vi "Main.vi"() -> ()   [LabVIEW 2022 SP3]
doc: "该范例项目基于标准状态机模板创建，演示用于采集、分析和显示数据的应用程序创建方法。 该应用程序的功能包括：显示配置对话框、在多次执行间保持设置、加载和保存数据，以及导出图像和文本文件。\n\n既不允许在采集过程中更新屏幕，也不允许将数据连续写入磁盘，因此特别适用于快速采集数据。"
uses:
  controls/State.ctl
  controls/Data.ctl
  controls/UI References.ctl
  controls/Graph Data.ctl
  <vilib>/Utility/miscctls.llb/LVAnnotationListTypeDef.ctl
  <vilib>/Utility/miscctls.llb/LVCursorListTypeDef.ctl
  controls/User Specified Data.ctl
  controls/HW Configuration.ctl
  controls/Simulated Signal Type.ctl
  controls/Analysis Configuration.ctl
  controls/New Data Behavior.ctl
  subVIs/Settings Dialog.vi
panel:
  in  "设置":bool
  in  "快照":bool
  in  "分析":bool
  in  "清空":bool
  in  "退出":bool
  in  "采集":bool
  in  "导出":bool
  in  "保存数据":bool
  in  "加载数据":bool
  out "图形":waveform(dbl)[](graph)
  out "状态栏":string
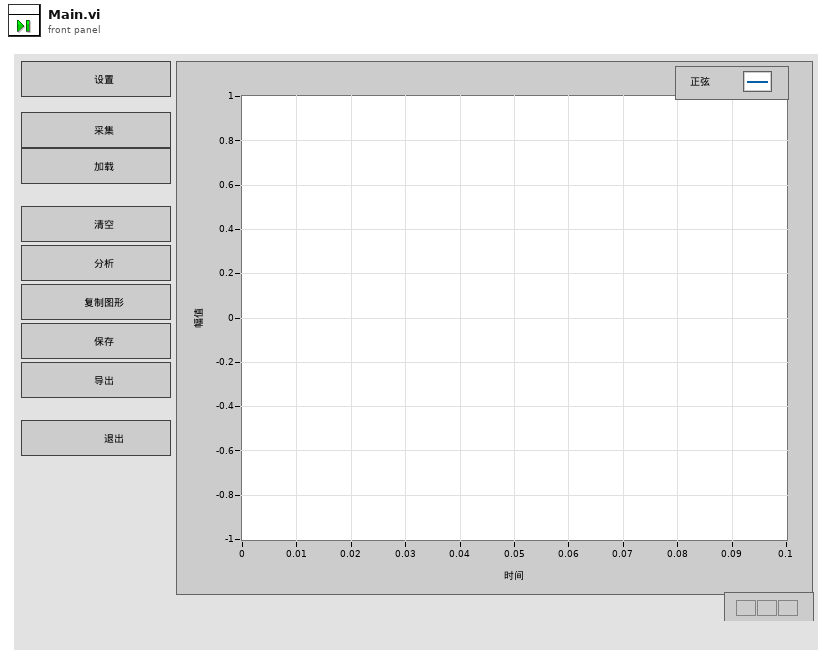
[diagram p1: front panel]
types:
  T1 = typedef "Data.ctl" = cluster{"UI引用":T2, "图形数据":T3, "用户定义":T6}
  T2 = typedef "UI References.ctl" = cluster{"退出引用":refnum<vi>, "保存引用":refnum<vi>, "打开引用":refnum<vi>, "导出引用":refnum<vi>, "采集引用":refnum<vi>, "配置引用":refnum<vi>, "图形引用":refnum<vi>, "清空引用":refnum<vi>, "分析引用":refnum<vi>, "状态引用":refnum<vi>, "快照引用":refnum<vi>}
  T3 = typedef "Graph Data.ctl" = cluster{"数据":waveform(dbl)[], "注释列表":T4, "游标列表":T5, "分析数据":waveform(dbl)[]}
  T4 = typedef "LVAnnotationListTypeDef.ctl" = cluster{"Name":string, "Color":u32, "Style":u8, "Point Style":u8, "Name Visible":bool, "Allow Drag":bool, "Annotation Mode":u32, "Plot":i32, "Index":i32, "Position":cluster{"X":dbl, "Y":dbl}, "X Scale":u32, "Y Scale":u32, "Show Arrow":bool, "Lock Name":bool, "Plot Area":i32, "Label Offset":cluster{"X":dbl, "Y":dbl}}[]
  T5 = typedef "LVCursorListTypeDef.ctl" = cluster{"Name":string, "Color":u32, "Style":u8, "Point Style":u8, "Name Visible":bool, "Allow Drag":bool, "Cursor Mode":u32, "Plot":i32, "Index":i32, "Position":cluster{"X":dbl, "Y":dbl}, "X Scale":u32, "Y Scale":u32, "Watch Plots":i32[], "Watch All Plots":bool, "Plot Area":i32, "Label Offset":cluster{"X":dbl, "Y":dbl}}[]
  T6 = typedef "User Specified Data.ctl" = cluster{"硬件配置":T7, "分析配置":T9, "新采集到数据时如何操作":T10}
  T7 = typedef "HW Configuration.ctl" = cluster{"硬件引用句柄<替换此项>":string, "信号类型<替换该项>":T8}
  T8 = typedef "Simulated Signal Type.ctl" = enum16{"Sine Wave", "Square Wave"}
  T9 = typedef "Analysis Configuration.ctl" = cluster{"统计":bool}
  T10 = typedef "New Data Behavior.ctl" = enum16{"Replace", "Overlay", "Append"}
  T11 = typedef "State.ctl" = enum16{"Initialize", "Wait for Event", "Update UI", "Configure", "Acquire", "Load Data", "Save Data", "Clear Data", "Export Data", "Analyze", "Copy Graph", "Exit"}
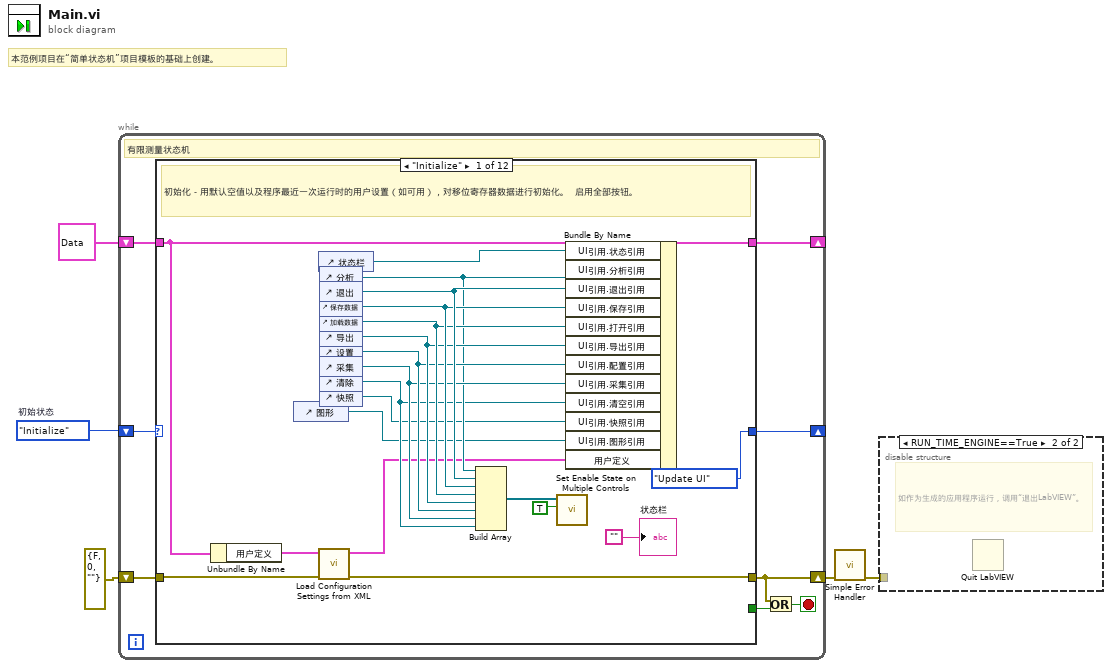
[diagram p0: block diagram]
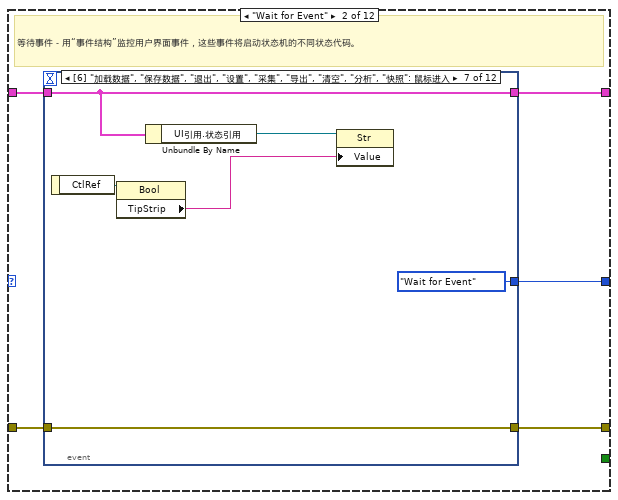
[diagram p3: hidden frame]
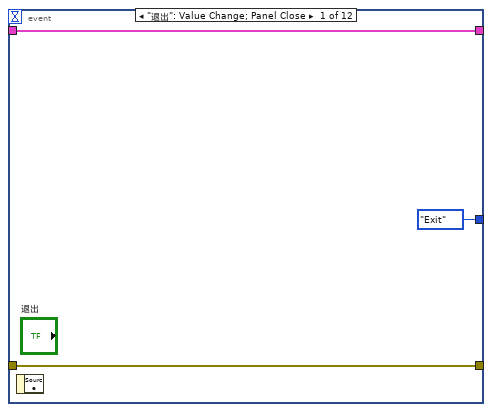
[diagram p4: hidden frame]
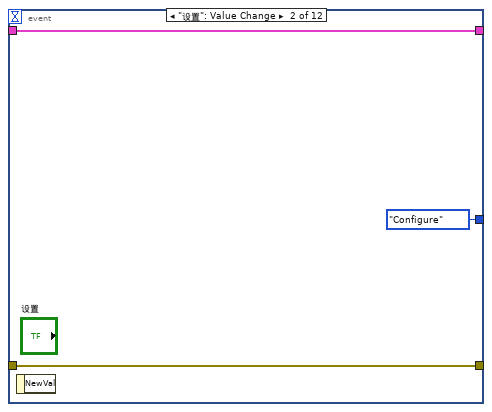
[diagram p5: hidden frame]
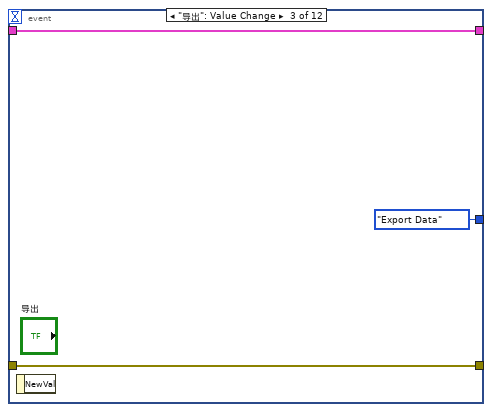
[diagram p6: hidden frame]
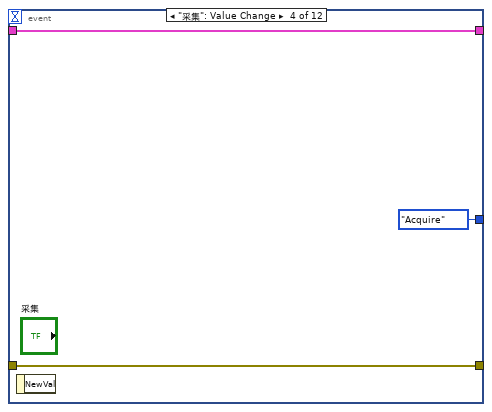
[diagram p7: hidden frame]
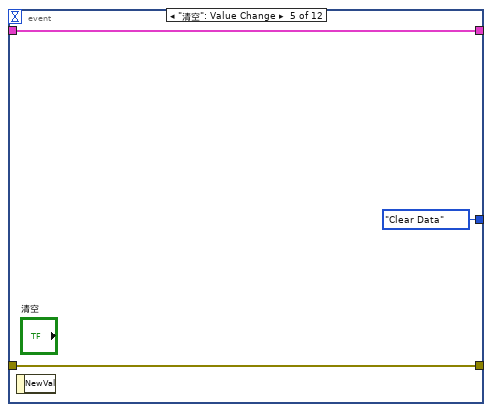
[diagram p8: hidden frame]
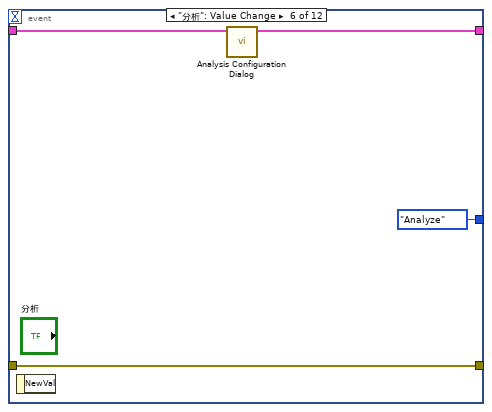
[diagram p9: hidden frame]
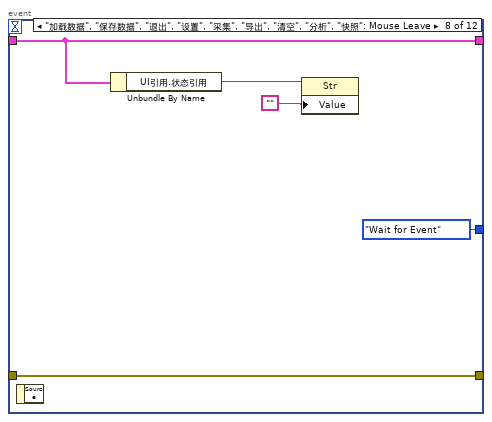
[diagram p10: hidden frame]
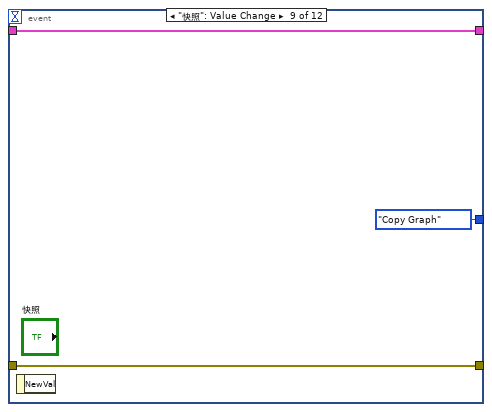
[diagram p11: hidden frame]
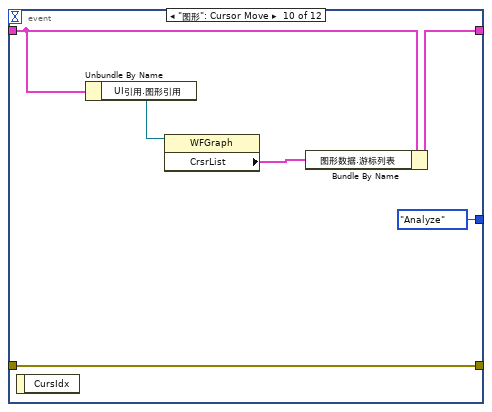
[diagram p12: hidden frame]
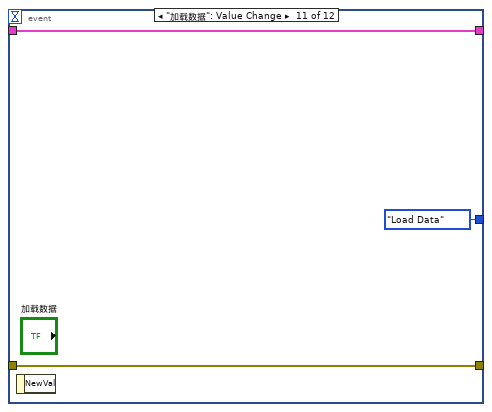
[diagram p13: hidden frame]
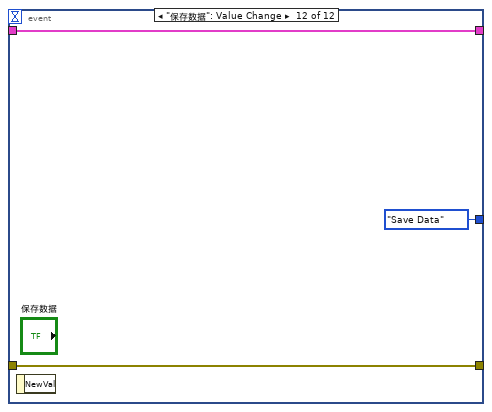
[diagram p14: hidden frame]
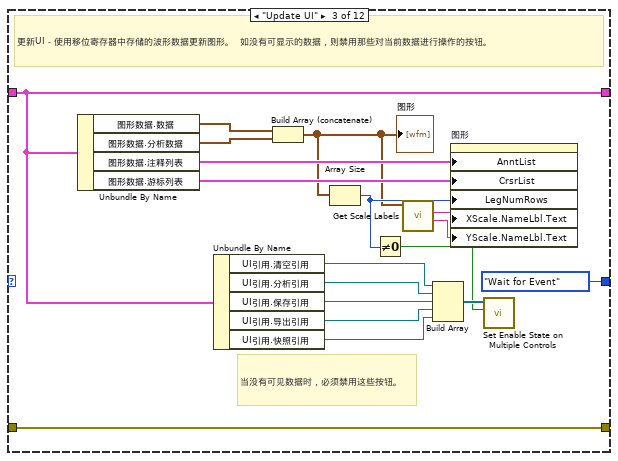
[diagram p15: hidden frame]
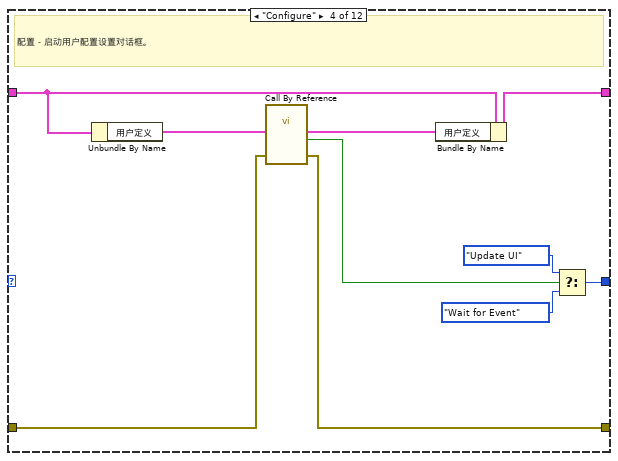
[diagram p16: hidden frame]
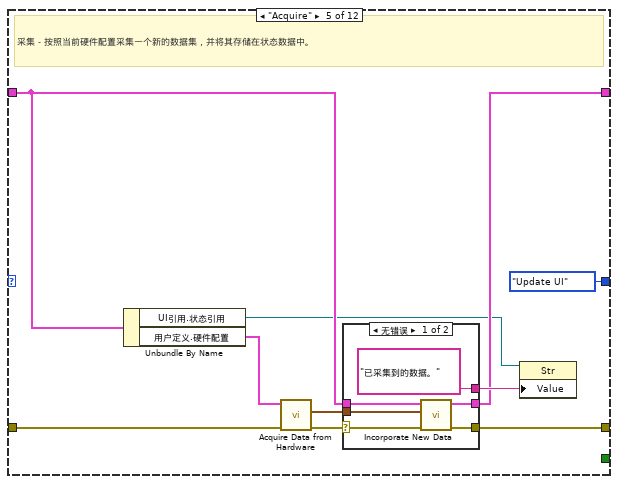
[diagram p17: hidden frame]
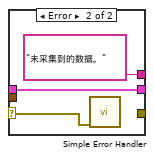
[diagram p18: hidden frame]
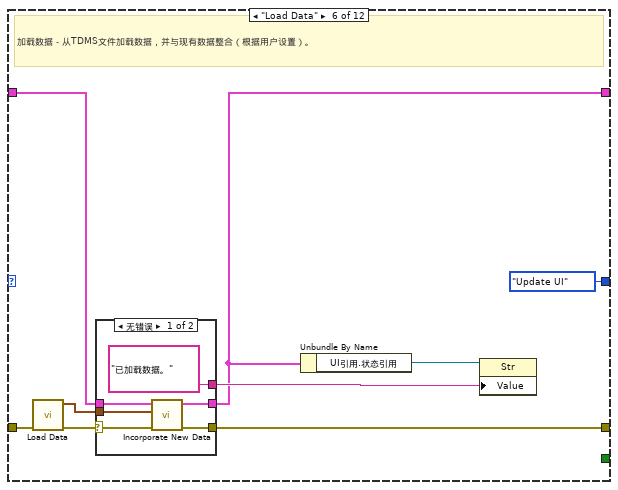
[diagram p19: hidden frame]
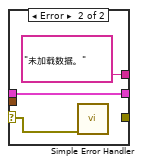
[diagram p20: hidden frame]
diagram:
  w5 = State."Initialize"  # 初始状态
  # "本范例项目在“简单状态机”项目模板的基础上创建。"
  n1 = while {
    shift-right: [w12] -> _
    shift-left: w5 -> [w13]
    shift-right: [w10] -> _
    shift-left: T1 {"UI引用"={"退出引用"=refnum, "保存引用"=refnum, "打开引用"=refnum, "导出引用"=refnum, "采集引用"=refnum, "配置引用"=refnum, "图形引用"=refnum, "清空引用"=refnum, "分析引用"=refnum, "状态引用"=refnum, "快照引用"=refnum}, "图形数据"={"数据"=[], "注释列表"=[], "游标列表"=[], "分析数据"=[]}, "用户定义"={"硬件配置"={"硬件引用句柄<替换此项>"="", "信号类型<替换该项>"=enum."Sine Wave"}, "分析配置"={"统计"=TRUE}, "新采集到数据时如何操作"=enum."Replace"}} ("Data") -> [w11]
    shift-right: [w6] -> w3
    shift-left: errorcluster {"status"=FALSE, "code"=0, "source"=""} ("error constant") -> [w9]
    stop <- w7 stop-if-true
    # "有限测量状态机"
    n2 = case shown="\"Initialize\"" w13 {
      tunnel: [State."Update UI" ("Next State") w39 State."Wait for Event" ("(Value Not Used)") w106 State."Update UI" ("Next State") State."Update UI" ("(Value Not Used)") State."Wait for Event" ("(Value Not Used)") State."Wait for Event" ("(Value Not Used)") State."Update UI" ("(Value Not Used)") State."Update UI" ("(Value Not Used)") State."Wait for Event" ("(Value Not Used)") w194] -> w12
      tunnel: [_ _ _ _ _ _ _ _ _ _ _ w193] -> w8
      tunnel: w11 -> [w25 w38 w99 w112 w118 w140 w153 w165 w176 w179 w185 w191]
      tunnel: [w33 w37 w99 w111 w117 w134 w153 w165 w175 w179 w185 w191] -> w10
      tunnel: w9 -> [w23 w36 w102 w110 w120 w139 w155 w168 w178 w180 w184 w188]
      tunnel: [w22 w35 w102 w109 w113 w138 w151 w162 w178 w180 w183 w187] -> w6
      frame "Initialize" {
        # "初始化－用默认空值以及程序最近一次运行时的用户设置（如可用），对移位寄存器数据进行初始化。  启用全部按钮。"
        n3 = Unbundle By Name(w25) -> ("用户定义"=w24:T6)
        n4 = control-ref of="图形"() -> (w14:refnum<vi>)
        n5 = control-ref of="状态栏"() -> (w20:refnum<vi>)
        n6 = call "Load Configuration Settings from XML.vi"("error in (no error)"=w23, "用户配置输入"=w24) -> ("error out"=w22:cluster{"状态":bool, "代码":i32, "源":string}, "用户配置输出"=w17:T6)  [unwired: 8 in]
        n7 = control-ref of="分析"() -> (w21:refnum<vi>)
        n8 = control-ref of="退出"() -> (w32:refnum<vi>)
        n9 = control-ref of="保存数据"() -> (w31:refnum<vi>)
        n10 = control-ref of="加载数据"() -> (w30:refnum<vi>)
        n11 = control-ref of="导出"() -> (w29:refnum<vi>)
        n12 = control-ref of="设置"() -> (w28:refnum<vi>)
        n13 = control-ref of="采集"() -> (w27:refnum<vi>)
        n14 = control-ref of="清除"() -> (w19:refnum<vi>)
        n15 = control-ref of="快照"() -> (w15:refnum<vi>)
        n16 = Build Array(w21, w32, w31, w30, w29, w28, w27, w19) -> (w26:refnum<vi>[])
        n17 = call "Set Enable State on Multiple Controls.vi"("启用？"=TRUE ("Enable?"), "控件"=w26) -> ()  [unwired: 10 in]
        n18 = Bundle By Name(cluster=w25, "UI引用.状态引用"=w20, "UI引用.分析引用"=w21, "UI引用.退出引用"=w32, "UI引用.保存引用"=w31, "UI引用.打开引用"=w30, "UI引用.导出引用"=w29, "UI引用.配置引用"=w28, "UI引用.采集引用"=w27, "UI引用.清空引用"=w19, "UI引用.快照引用"=w15, "UI引用.图形引用"=w14, "用户定义"=w17) -> (w33:T1)
        "状态栏" <- "" ("Status Bar")
      }
      frame "Wait for Event" {
        # "等待事件－用“事件结构”监控用户界面事件，这些事件将启动状态机的不同状态代码。"
        n19 = event shown="[6] \"加载数据\", \"保存数据\", \"退出\", \"设置\", \"采集\", \"导出\", \"清空\", \"分析\", \"快照\": 鼠标进入" {
          selector: _ -> [_ _ _ _ _ _ _ _ _ _ _ _]
          dyn-events: _ -> [_ _ _ _ _ _ _ _ _ _ _ _]
          timeout: _ -> [_ _ _ _ _ _ _ _ _ _ _ _]
          tunnel: [State."Exit" ("Next State") State."Configure" ("Next State") State."Export Data" ("Next State") State."Acquire" ("Next State") State."Clear Data" ("Next State") State."Analyze" ("Next State") State."Wait for Event" ("Next State") State."Wait for Event" ("Next State") State."Copy Graph" ("Next State") State."Analyze" ("Next State") State."Load Data" ("Next State") State."Save Data" ("Next State")] -> w39
          tunnel: w38 -> [w41 w45 w48 w51 w54 w56 w62 w68 w72 w73 w80 w83]
          tunnel: [w41 w45 w48 w51 w54 w55 w62 w68 w72 w76 w80 w83] -> w37
          tunnel: w36 -> [w40 w44 w47 w50 w53 w58 w64 w69 w71 w78 w79 w82]
          tunnel: [w40 w44 w47 w50 w53 w58 w64 w69 w71 w78 w79 w82] -> w35
          event "退出": Value Change; Panel Close {
            n20 = event-data() -> ()  [unwired: 1 in, 1 out]
          }
          event "设置": Value Change {
            n21 = event-data() -> ()  [unwired: 1 in, 1 out]
          }
          event "导出": Value Change {
            n22 = event-data() -> ()  [unwired: 1 in, 1 out]
          }
          event "采集": Value Change {
            n23 = event-data() -> ()  [unwired: 1 in, 1 out]
          }
          event "清空": Value Change {
            n24 = event-data() -> ()  [unwired: 1 in, 1 out]
          }
          event "分析": Value Change {
            n25 = event-data() -> ()  [unwired: 1 in, 1 out]
            n26 = call "Analysis Configuration Dialog.vi"("数据输入"=w56) -> ("数据输出"=w55:T1)  [unwired: 10 in]
          }
          event "加载数据", "保存数据", "退出", "设置", "采集", "导出", "清空", "分析", "快照": Mouse Enter {
            n27 = event-data() -> ("CtlRef"=w63:refnum<vi>)  [unwired: 1 in]
            n28 = property on="Property Node" class="Bool"(reference=w63) -> ("TipStrip"=w60:string)  [unwired: 1 in, 2 out]
            n29 = Unbundle By Name(w62) -> ("UI引用.状态引用"=w61:refnum<vi>)
            n30 = property on="Property Node" class="Str"(reference=w61, "Value"=w60) -> ()  [unwired: 1 in, 2 out]
          }
          event "加载数据", "保存数据", "退出", "设置", "采集", "导出", "清空", "分析", "快照": Mouse Leave {
            n31 = event-data() -> ()  [unwired: 1 in, 1 out]
            n32 = Unbundle By Name(w68) -> ("UI引用.状态引用"=w67:refnum<vi>)
            n33 = property on="Property Node" class="Str"(reference=w67, "Value"="") -> ()  [unwired: 1 in, 2 out]
          }
          event "快照": Value Change {
            n34 = event-data() -> ()  [unwired: 1 in, 1 out]
          }
          event "图形": Cursor Move {
            n35 = event-data() -> ()  [unwired: 1 in, 1 out]
            n36 = Unbundle By Name(w73) -> ("UI引用.图形引用"=w75:refnum<vi>)
            n37 = property on="Property Node" class="WFGraph"(reference=w75) -> ("CrsrList"=w74:T5)  [unwired: 1 in, 2 out]
            n38 = Bundle By Name(cluster=w73, "图形数据.游标列表"=w74) -> (w76:T1)
          }
          event "加载数据": Value Change {
            n39 = event-data() -> ()  [unwired: 1 in, 1 out]
          }
          event "保存数据": Value Change {
            n40 = event-data() -> ()  [unwired: 1 in, 1 out]
          }
        }
      }
      frame "Update UI" {
        # "当没有可见数据时，必须禁用这些按钮。"
        # "更新UI－使用移位寄存器中存储的波形数据更新图形。  如没有可显示的数据，则禁用那些对当前数据进行操作的按钮。"
        n41 = Unbundle By Name(w99) -> ("图形数据.数据"=w95:waveform(dbl)[], "图形数据.分析数据"=w85:waveform(dbl)[], "图形数据.注释列表"=w100:T4, "图形数据.游标列表"=w96:T5)
        n42 = Unbundle By Name(w99) -> ("UI引用.清空引用"=w91:refnum<vi>, "UI引用.分析引用"=w90:refnum<vi>, "UI引用.保存引用"=w98:refnum<vi>, "UI引用.导出引用"=w88:refnum<vi>, "UI引用.快照引用"=w89:refnum<vi>)
        n43 = Build Array (concatenate)(w95, w85) -> (w93:waveform(dbl)[])
        "图形" <- w93
        n44 = Array Size(array=w93) -> (size(s)=w94:i32)
        n45 = Not Equal To 0?(x=w94) -> (x != 0?=w92:bool)
        n46 = call "Get Scale Labels.vi"("波形数组"=w93) -> ("Y标尺标签文本"=w86:string, "X标尺标签文本"=w87:string)  [unwired: 9 in]
        n47 = Build Array(w91, w90, w98, w88, w89) -> (w97:refnum<vi>[])
        n48 = property on="图形" class="WFGraph (严格)"("AnntList"=w100, "CrsrList"=w96, "LegNumRows"=w94, "XScale.NameLbl.Text"=w87, "YScale.NameLbl.Text"=w86) -> ()  [unwired: 2 in, 2 out]
        n49 = call "Set Enable State on Multiple Controls.vi"("启用？"=w92, "控件"=w97) -> ()  [unwired: 10 in]
      }
      frame "Configure" {
        # "配置－启动用户配置设置对话框。"
        n50 = Unbundle By Name(w112) -> ("用户定义"=w104:T6)
        n51 = call-by-ref "?"("error in (no error)"=w110, "配置输入"=w104) -> ("error out"=w109:cluster{"状态":bool, "代码":i32, "源":string}, "需要刷新UI？"=w108:bool, "配置输出"=w103:T6)  [unwired: 9 in, 2 out]
        n52 = Bundle By Name(cluster=w112, "用户定义"=w103) -> (w111:T1)
        n53 = Select(t=State."Update UI" ("Next State if true"), s=w108, f=State."Wait for Event" ("Next State if false")) -> (s? t:f=w106:T11)
      }
      frame "Acquire" {
        # "采集－按照当前硬件配置采集一个新的数据集，并将其存储在状态数据中。"
        n54 = Unbundle By Name(w118) -> ("UI引用.状态引用"=w114:refnum<vi>, "用户定义.硬件配置"=w121:T7)
        n55 = call "Acquire Data from Hardware.vi"("error in (no error)"=w120, "硬件配置"=w121) -> ("error out"=w115:cluster{"状态":bool, "代码":i32, "源":string}, "图形数据"=w116:waveform(dbl)[])  [unwired: 8 in]
        n56 = case shown="无错误" w115 {
          selector: w115 -> [w125 w130]
          tunnel: w118 -> [w124 w131]
          tunnel: [w128 w131] -> w117
          tunnel: [w127 _] -> w113
          tunnel: w116 -> [w126 _]
          tunnel: ["已采集到的数据。" ("Data acquired") "未采集到的数据。" ("Data not acquired")] -> w119
          frame No Error {
            n57 = call "Incorporate New Data.vi"("error in (no error)"=w125, "新图形数据"=w126, "数据输入"=w124) -> ("error out"=w127:cluster{"状态":bool, "代码":i32, "源":string}, "数据输出"=w128:T1)  [unwired: 7 in]
          }
          frame Error {
            n58 = call <vilib>:"Simple Error Handler.vi"("error in (no error)"=w130) -> ()  [unwired: 4 in, 5 out]
          }
        }
        n59 = property on="Property Node" class="Str"(reference=w114, "Value"=w119) -> ()  [unwired: 1 in, 2 out]
      }
      frame "Load Data" {
        # "加载数据－从TDMS文件加载数据，并与现有数据整合（根据用户设置）。"
        n60 = call "Load Data.vi"("error in (no error)"=w139) -> ("error out"=w136:cluster{"状态":bool, "代码":i32, "源":string}, "新图形数据"=w133:waveform(dbl)[])  [unwired: 9 in]
        n61 = case shown="无错误" w136 {
          selector: w136 -> [w143 w148]
          tunnel: w140 -> [w142 w149]
          tunnel: [w146 w149] -> w134
          tunnel: [w145 _] -> w138
          tunnel: w133 -> [w144 _]
          tunnel: ["已加载数据。" ("Data loaded") "未加载数据。" ("Data not loaded")] -> w135
          frame No Error {
            n62 = call "Incorporate New Data.vi"("error in (no error)"=w143, "新图形数据"=w144, "数据输入"=w142) -> ("error out"=w145:cluster{"状态":bool, "代码":i32, "源":string}, "数据输出"=w146:T1)  [unwired: 7 in]
          }
          frame Error {
            n63 = call <vilib>:"Simple Error Handler.vi"("error in (no error)"=w148) -> ()  [unwired: 4 in, 5 out]
          }
        }
        n64 = Unbundle By Name(w134) -> ("UI引用.状态引用"=w132:refnum<vi>)
        n65 = property on="Property Node" class="Str"(reference=w132, "Value"=w135) -> ()  [unwired: 1 in, 2 out]
      }
      frame "Save Data" {
        # "保存数据－将现有的测量数据保存为TDMS文件。"
        n66 = Unbundle By Name(w153) -> ("UI引用.状态引用"=w152:refnum<vi>, "图形数据.数据"=w156:waveform(dbl)[])
        n67 = call "Save Data.vi"("error in (no error)"=w155, "数据"=w156) -> ("error out"=w154:cluster{"状态":bool, "代码":i32, "源":string})  [unwired: 9 in]
        n68 = case shown="无错误" w154 {
          selector: w154 -> [w158 w161]
          tunnel: ["已保存数据。" ("Data saved") "未保存数据。" ("Data not saved")] -> w150
          tunnel: [w158 _] -> w151
          frame No Error {
          }
          frame Error {
            n69 = call <vilib>:"Simple Error Handler.vi"("error in (no error)"=w161) -> ()  [unwired: 4 in, 5 out]
          }
        }
        n70 = property on="Property Node" class="Str"(reference=w152, "Value"=w150) -> ()  [unwired: 1 in, 2 out]
      }
      frame "Export Data" {
        # "导出数据－将当前已加载的测量和分析数据导出至文本文件，以便导入电子表格或其他应用程序。"
        n71 = Unbundle By Name(w165) -> ("UI引用.状态引用"=w163:refnum<vi>, "图形数据"=w164:T3)
        n72 = call "Export Data.vi"("error in (no error)"=w168, "图形数据"=w164) -> ("error out"=w166:cluster{"状态":bool, "代码":i32, "源":string})  [unwired: 9 in]
        n73 = case shown="无错误" w166 {
          selector: w166 -> [w170 w173]
          tunnel: ["已导入数据。" ("Data exported") "未导入数据。" ("Data not exported")] -> w167
          tunnel: [w170 _] -> w162
          frame No Error {
          }
          frame Error {
            n74 = call <vilib>:"Simple Error Handler.vi"("error in (no error)"=w173) -> ()  [unwired: 4 in, 5 out]
          }
        }
        n75 = property on="Property Node" class="Str"(reference=w163, "Value"=w167) -> ()  [unwired: 1 in, 2 out]
      }
      frame "Clear Data" {
        # "清空数据－清空当前图形中的数据。"
        n76 = Bundle By Name(cluster=w176, "图形数据"=T3 {"数据"=[], "注释列表"=[], "游标列表"=[], "分析数据"=[]} ("Graph")) -> (w175:T1)
      }
      frame "Analyze" {
        # "#推荐代码 - 在此处添加自定义信号分析。"
        # "分析－分析测量数据。"
        n77 = Unbundle By Name(w179) -> ("图形数据"=w181:T3)
        n78 = call "Statistical Analysis.vi"("图形数据输入"=w181) -> ()  [unwired: 9 in, 2 out]
      }
      frame "Copy Graph" {
        # "复制图像－在剪贴板中存放图形图像，以便粘贴至报表或email。"
        n79 = call "Copy Graph to Clipboard.vi"("error in (no error)"=w184, "图形数据"=w185) -> ("error out"=w183:cluster{"状态":bool, "代码":i32, "源":string})  [unwired: 9 in]
      }
      frame "Exit" {
        w193 = TRUE  # 停止循环？
        w194 = State."Exit"  # （未用值）
        # "退出－将用户设置保存为XML文件并停止执行。"
        n80 = Unbundle By Name(w191) -> ("UI引用.状态引用"=w189:refnum<vi>, "用户定义"=w192:T6)
        n81 = call "Save Configuration Settings to XML.vi"("error in (no error)"=w188, "用户配置"=w192) -> ("error out"=w187:cluster{"状态":bool, "代码":i32, "源":string})  [unwired: 9 in]
        n82 = property on="Property Node" class="Str"(reference=w189, "Value"="应用程序退出。" ("Stopped")) -> ()  [unwired: 1 in, 2 out]
      }
    }
    n83 = Or(x=w6, y=w8) -> (x .or. y?=w7:bool)
  }
  n84 = call <vilib>:"Simple Error Handler.vi"("error in (no error)"=w3) -> ("error out"=w1:errorcluster)  [unwired: 4 in, 4 out]
  n85 = disable-structure "Conditional Disable Structure" shown="RUN_TIME_ENGINE==True" {
    disable-tunnel: w1 -> [_ _]
    frame condition #0 (active) {
    }
    frame condition #1 {
      # "如作为生成的应用程序运行，调用“退出LabVIEW”。"
      n86 = Quit LabVIEW() -> ()  [unwired: 1 in]
    }
  }
